vi "Test-Motors with Encoders-Report Motor State.vi"() -> ()   [LabVIEW 2014, in "Comp Motors with Encoders.lvlib"]
uses:
  Comp Motors with Encoders.lvlib
  Robot Actor Framework/Trace/Trace Controller Class/Config.ctl
  Robot/Joystick/Joystick Class/Joystick State.ctl
  Robot/Joystick/Joystick Class/Button State.ctl
  Robot/Joystick/Joystick Class/Axis State.ctl
  Comp Xbox One Controller/Comp XBox One Controller Class/Comp X1 Config.ctl
  <vilib>/Rock Robotics/WPI/Joystick/WPI_JoystickDeviceEnum.ctl
  Comp Trace Controller/Comp Trace Controller Class/Comp Trace Controller.lvclass
  Comp Pressure/Comp Pressure Class/Comp Pressure.lvclass
  Comp Xbox One Controller/Comp XBox One Controller Class/Comp XBox One Controller.lvclass
  Comp Xbox One Controller/Test-XBox Controller-Receive Updates/Test-XBox Controller-Receive Updates.lvclass
  Comp Xbox One Controller/Comp XBox One Controller Class/Comp XBox One Controller.lvclass/Comp XBox One Controller.ctl
  <vilib>/Rock Robotics/WPI/DriverStation/WPI_DriverStationRobotMode2.ctl
  Comp Xbox One Controller/Test-XBox Controller-Receive Updates Messages/Receive Joystick Update Msg/Receive Joystick Update Msg.lvclass
  Robot/Joystick/Joystick Messages/Request Joystick State Msg/Request Joystick State Msg.lvclass/Request Joystick State Msg.ctl
  <vilib>/ActorFramework/Message Enqueuer/Message Enqueuer.lvclass/Message Enqueuer.ctl
  <vilib>/ActorFramework/Message Enqueuer/Enqueue.vi
  <vilib>/ActorFramework/Message Priority Queue/Priority Enqueue.vi
  Robot/Joystick/Joystick Messages/Request Joystick State Msg/Request Joystick State Msg.lvclass
  <vilib>/ActorFramework/Stop Msg/Stop Msg.lvclass
  <vilib>/ActorFramework/Actor/Actor.lvclass
  Robot Actor Framework/Trace/Trace Controller Class/Trace Controller.lvclass
  Robot/Joystick/Joystick Class/Joystick.lvclass
panel:
  in  "XBox One Controller Config":T1={"Joystick USB"=enum."USB 0", "Deadband"=0.1}
  in  "Joystick State":T3
  in  "Test Loop":u32=75
  out "Enable Tele":bool caption="Enabled Teleop"
  in  "Stop Test Loop 1":bool=TRUE
  in  "Finish Test":bool=TRUE
  in  "Start Test":bool=TRUE
  in  "Trace Controller Config":T6={"Folder Pattern"="/media/sd%s1", "Starting Letter Position"=1, "Min Free Space (MB)"=50.0, "Max Folders to Check"=10, "Trace Level"=enum."Debug"} {"Min Free Space (MB)" format="%#_13g"}
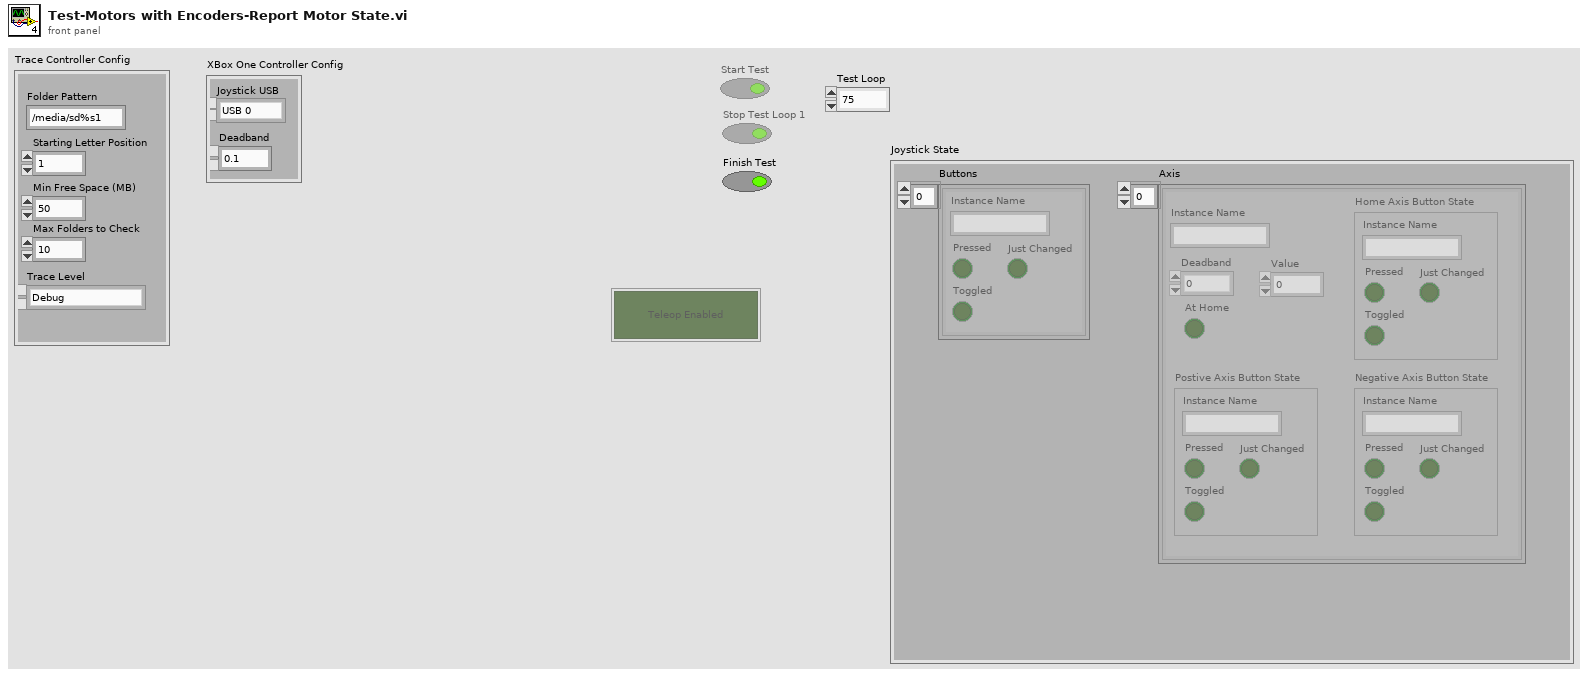
[diagram p1: front panel]
types:
  T1 = typedef "Comp XBox One Controller.lvlib/Comp XBox One Controller.lvclass/Comp X1 Config.ctl" = cluster{"Joystick USB":T2, "Deadband":dbl}
  T2 = typedef "WPI_JoystickDeviceEnum.ctl" = enum16{"USB 0", "USB 1", "USB 2", "USB 3", "USB 4", "USB 5"}
  T3 = typedef "Joystick.lvlib/Joystick.lvclass/Joystick State.ctl" = cluster{"Buttons":T4[], "Axis":T5[]}
  T4 = typedef "Joystick.lvlib/Joystick.lvclass/Button State.ctl" = cluster{"Pressed":bool, "Instance Name":string, "Toggled":bool, "Just Changed":bool}
  T5 = typedef "Joystick.lvlib/Joystick.lvclass/Axis State.ctl" = cluster{"Instance Name":string, "Deadband":dbl, "Value":dbl, "At Home":bool, "Postive Axis Button State":T4, "Negative Axis Button State":T4, "Home Axis Button State":T4}
  T6 = typedef "Robot Actor Framework.lvlib/Trace.lvlib/Trace Controller.lvclass/Config.ctl" = cluster{"Folder Pattern":string, "Starting Letter Position":i32, "Min Free Space (MB)":dbl, "Max Folders to Check":u32, "Trace Level":enum16{"Critical", "Error", "Warning", "Informational", "Debug"}}
  T7 = enum16{"Critical", "Error", "Warning", "Informational", "Debug"}
  T8 = enum8{"Enabled", "Disabled", "Disabled and Grayed Out"}
  T9 = typedef "WPI_DriverStationRobotMode2.ctl" = enum16{"Autonomous Disabled", "Autonomous Enabled", "Teleop Disabled", "Teleop Enabled", "Disconnected", "Finish", "Test Disabled", "Test Enabled", "Emergency Stopped"}
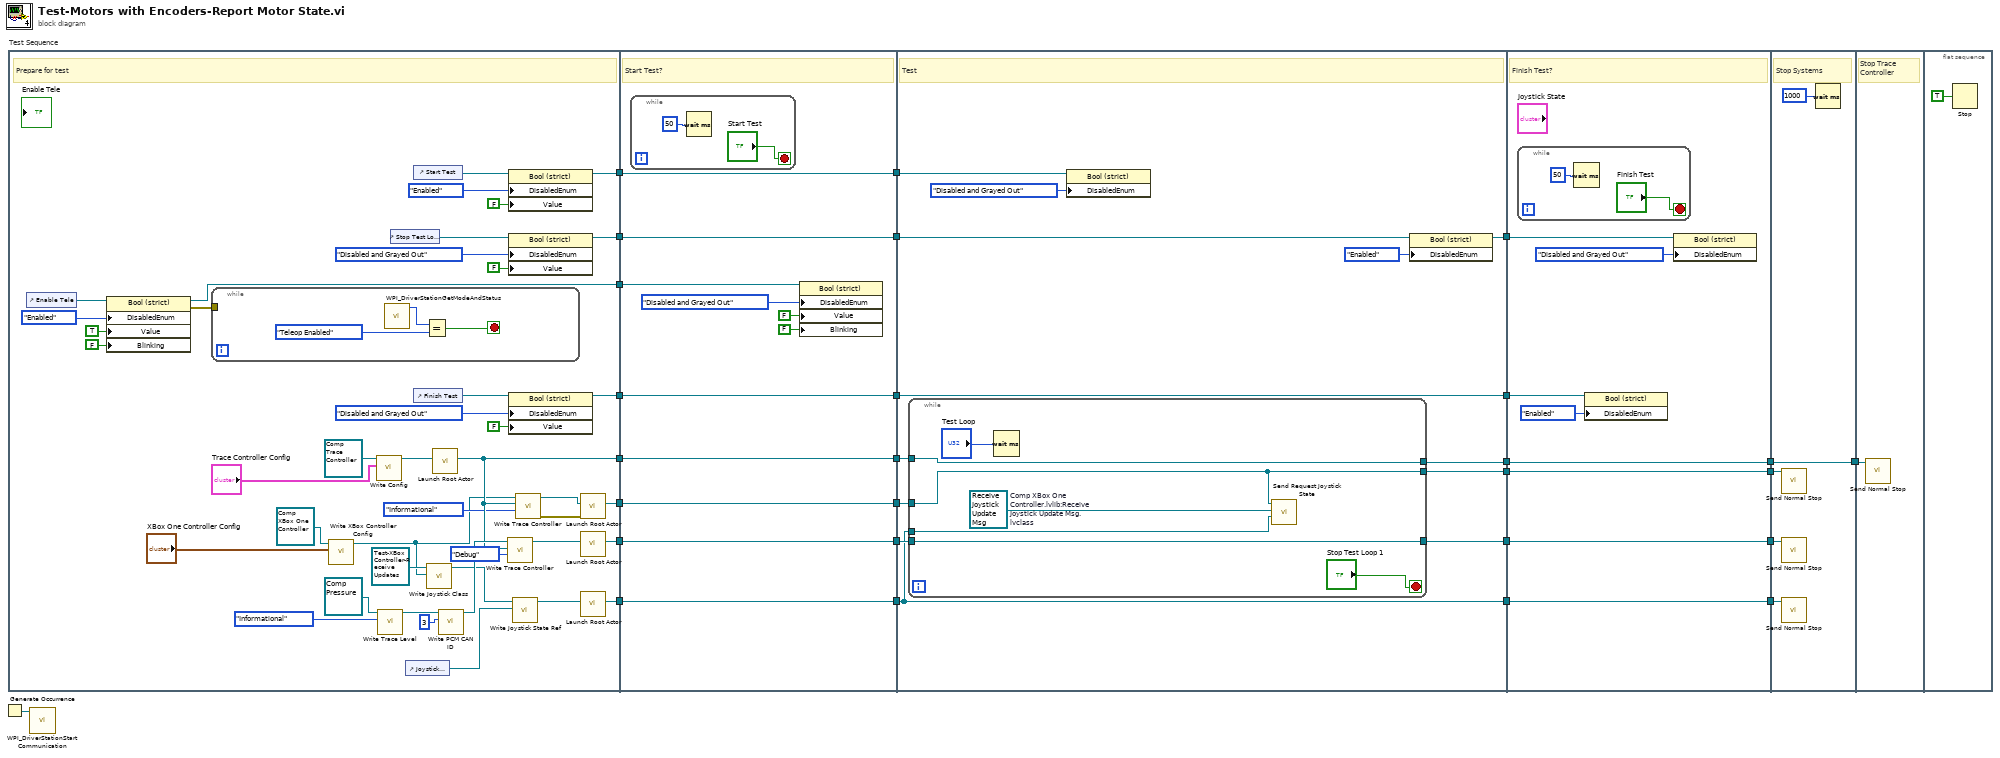
[diagram p0: block diagram]
diagram:
  n1 = Generate Occurrence() -> (w27:refnum<k4>)
  n2 = flat-sequence "Test Sequence" {
    tunnel: [w57] -> w16
    tunnel: [w59] -> w15
    tunnel: [w58] -> w14
    tunnel: [w47] -> w13
    tunnel: [w46] -> w11
    tunnel: [w45] -> w6
    tunnel: [w39] -> w5
    tunnel: [w29] -> w3
    tunnel: [w83] -> w19
    tunnel: [w82] -> w18
    tunnel: [w81] -> w17
    tunnel: w16 -> [w83]
    tunnel: w15 -> [w82]
    tunnel: w14 -> [w81]
    tunnel: w13 -> [w80]
    tunnel: [w80] -> w12
    tunnel: w11 -> [w79]
    tunnel: [w79] -> w10
    tunnel: [w78] -> w7
    tunnel: w6 -> [w78]
    tunnel: w5 -> [w77]
    tunnel: [w73] -> w4
    tunnel: w3 -> [w73]
    tunnel: [w93] -> w22
    tunnel: [w95] -> w21
    tunnel: [w94] -> w20
    tunnel: w19 -> [w98]
    tunnel: w18 -> [w96]
    tunnel: w17 -> [w97]
    tunnel: w12 -> [w92]
    tunnel: w10 -> [w90]
    tunnel: [w88] -> w9
    tunnel: [w87] -> w8
    tunnel: w7 -> [w87]
    tunnel: w4 -> [w86]
    tunnel: [w86] -> w2
    tunnel: [w113] -> w25
    tunnel: [w112] -> w24
    tunnel: [w111] -> w23
    tunnel: w22 -> [w113]
    tunnel: w21 -> [w112]
    tunnel: w20 -> [w111]
    tunnel: w9 -> [w110]
    tunnel: w8 -> [w107]
    tunnel: w2 -> [w106]
    tunnel: [w106] -> w1
    tunnel: [w120] -> w26
    tunnel: w25 -> [w120]
    tunnel: w24 -> [w119]
    tunnel: w23 -> [w117]
    tunnel: w1 -> [w116]
    tunnel: w26 -> [w121]
    frame #0 {
      # "Prepare for test"
      n3 = control-ref of="Enable Tele"() -> (w44:refnum<vi>)
      n4 = property class="Bool (strict)"(reference=w44, "DisabledEnum"=T8."Enabled" ("Disabled"), "Value"=TRUE, "Blinking"=FALSE) -> (reference out=w39:refnum<vi>, error out=w41:errorcluster)  [unwired: 1 in]
      n5 = while {
        tunnel: w41 -> [_]
        stop <- w70 stop-if-true
        n6 = call <vilib>:"WPI_DriverStationGetModeAndStatus.vi"() -> ("Robot Mode"=w72:T9)  [unwired: 10 in, 1 out]
        n7 = Equal?(x=w72, y=WPI_DriverStationRobotMode2."Teleop Enabled") -> (x = y?=w70:bool)
      }
      n8 = call "Write XBox Controller Config.vi"("XBox One Controller Config"="XBox One Controller Config", "Comp XBox One Controller in"=refnum<class "Comp XBox One Controller.lvclass"> refnum ("Comp XBox One Controller.lvlib:Comp XBox One Controller.lvclass")) -> ("Comp XBox One Controller out"=w31:refnum<class "Comp XBox One Controller.lvclass">)  [unwired: 8 in, 1 out]
      n9 = call-dynamic "Write Config.vi"("Config"="Trace Controller Config", "Trace Controller in"=refnum<class "Comp Trace Controller.lvclass"> refnum ("Comp Trace Controller.lvlib:Comp Trace Controller.lvclass")) -> ("Trace Controller out"=w62:refnum<class "Comp Trace Controller.lvclass">)  [unwired: 8 in, 1 out]
      n10 = call-dynamic "Write Trace Level.vi"("Trace Level"=T7."Informational", "System Actor in"=refnum<class "Comp Pressure.lvclass"> refnum ("Comp Pressure.lvlib:Comp Pressure.lvclass")) -> ("System Actor out"=w67:refnum<class "Comp Pressure.lvclass">)  [unwired: 8 in, 1 out]
      n11 = control-ref of="Stop Test Loop 1"() -> (w51:refnum<vi>)
      n12 = control-ref of="Joystick State"() -> (w33:refnum<vi>)
      n13 = control-ref of="Start Test"() -> (w56:refnum<vi>)
      n14 = control-ref of="Finish Test"() -> (w50:refnum<vi>)
      n15 = call-dynamic "Write Joystick Class.vi"("Joystick.lvlib:Joystick.lvclass"=w31, "Test-XBox Controller-Receive Updates in"=refnum<class "Test-XBox Controller-Receive Updates.lvclass"> refnum ("Comp XBox One Controller.lvlib:Test-XBox Controller-Receive Updates.lvclass")) -> ("Test-XBox Controller-Receive Updates out"=w34:refnum<class "Test-XBox Controller-Receive Updates.lvclass">)  [unwired: 8 in, 1 out]
      n16 = call <vilib>:"Launch Root Actor.vi"("Actor"=w62) -> ("Actor's Enqueuer"=w58:refnum<class "Message Enqueuer.lvclass">)  [unwired: 9 in, 1 out]
      n17 = call-dynamic "Write PCM CAN ID.vi"("PCM CAN ID"=u8 3, "Comp Pressure in"=w67) -> ("Comp Pressure out"=w68:refnum<class "Comp Pressure.lvclass">)  [unwired: 8 in, 1 out]
      n18 = call-dynamic "Write Trace Controller.vi"("Trace Level"=T7."Debug", "Trace Controller"=w58, "System Actor in"=w68) -> ("System Actor out"=w69:refnum<class "Comp Pressure.lvclass">)  [unwired: 7 in, 1 out]
      n19 = property class="Bool (strict)"(reference=w56, "DisabledEnum"=T8."Enabled" ("Disabled"), "Value"=FALSE) -> (reference out=w47:refnum<vi>)  [unwired: 1 in, 1 out]
      n20 = property class="Bool (strict)"(reference=w51, "DisabledEnum"=T8."Disabled and Grayed Out" ("Disabled"), "Value"=FALSE) -> (reference out=w46:refnum<vi>)  [unwired: 1 in, 1 out]
      n21 = property class="Bool (strict)"(reference=w50, "DisabledEnum"=T8."Disabled and Grayed Out" ("Disabled"), "Value"=FALSE) -> (reference out=w45:refnum<vi>)  [unwired: 1 in, 1 out]
      n22 = call-dynamic "Write Joystick State Ref.vi"("Joystick State Ref"=w33, "Test-XBox Controller-Receive Updates in"=w34) -> ("Test-XBox Controller-Receive Updates out"=w32:refnum<class "Test-XBox Controller-Receive Updates.lvclass">)  [unwired: 8 in, 1 out]
      n23 = call-dynamic "Write Trace Controller.vi"("Trace Level"=T7."Informational", "Trace Controller"=w58, "System Actor in"=w31) -> ("error out"=w64:errorcluster, "System Actor out"=w63:refnum<class "Comp XBox One Controller.lvclass">)  [unwired: 7 in]
      n24 = call <vilib>:"Launch Root Actor.vi"("error in (no error)"=w64, "Actor"=w63) -> ("Actor's Enqueuer"=w57:refnum<class "Message Enqueuer.lvclass">)  [unwired: 8 in, 1 out]
      n25 = call <vilib>:"Launch Root Actor.vi"("Actor"=w69) -> ("Actor's Enqueuer"=w59:refnum<class "Message Enqueuer.lvclass">)  [unwired: 9 in, 1 out]
      n26 = call <vilib>:"Launch Root Actor.vi"("Actor"=w32) -> ("Actor's Enqueuer"=w29:refnum<class "Message Enqueuer.lvclass">)  [unwired: 9 in, 1 out]
    }
    frame #1 {
      # "Start Test?"
      n27 = while {
        stop <- "Start Test" stop-if-true
        n28 = Wait (ms)(milliseconds to wait=u32 50) -> ()  [unwired: 1 out]
      }
      n29 = property class="Bool (strict)"(reference=w77, "DisabledEnum"=T8."Disabled and Grayed Out" ("Disabled"), "Value"=FALSE, "Blinking"=FALSE) -> ()  [unwired: 1 in, 2 out]
    }
    frame #2 {
      # "Test"
      n30 = while {
        tunnel: w97 -> [w104]
        tunnel: [w104] -> w93
        tunnel: w98 -> [w101]
        tunnel: [w101] -> w95
        tunnel: w96 -> [w103]
        tunnel: [w103] -> w94
        tunnel: w86 -> [w100]
        stop <- "Stop Test Loop 1" stop-if-true
        w99 = refnum<class "Receive Joystick Update Msg.lvclass"> refnum  # Comp XBox One Controller.lvlib:Receive Joystick Update Msg.lvclass
        n31 = Wait (ms)(milliseconds to wait="Test Loop") -> ()  [unwired: 1 out]
        n32 = call "Send Request Joystick State.vi"("Caller Enqueuer"=w100, "Joystick State Msg"=w99, "Message Enqueuer"=w101) -> ()  [unwired: 7 in, 2 out]
      }
      n33 = property class="Bool (strict)"(reference=w92, "DisabledEnum"=T8."Disabled and Grayed Out" ("Disabled")) -> ()  [unwired: 1 in, 2 out]
      n34 = property class="Bool (strict)"(reference=w90, "DisabledEnum"=T8."Enabled" ("Disabled")) -> (reference out=w88:refnum<vi>)  [unwired: 1 in, 1 out]
    }
    frame #3 {
      # "Finish Test?"
      n35 = while {
        stop <- "Finish Test" stop-if-true
        n36 = Wait (ms)(milliseconds to wait=u32 50) -> ()  [unwired: 1 out]
      }
      n37 = property class="Bool (strict)"(reference=w107, "DisabledEnum"=T8."Enabled" ("Disabled")) -> ()  [unwired: 1 in, 2 out]
      n38 = property class="Bool (strict)"(reference=w110, "DisabledEnum"=T8."Disabled and Grayed Out" ("Disabled")) -> ()  [unwired: 1 in, 2 out]
    }
    frame #4 {
      # "Stop Systems"
      n39 = call <vilib>:"Send Normal Stop.vi"("Message Enqueuer"=w119) -> ()  [unwired: 10 in, 1 out]
      n40 = call <vilib>:"Send Normal Stop.vi"("Message Enqueuer"=w117) -> ()  [unwired: 10 in, 1 out]
      n41 = call <vilib>:"Send Normal Stop.vi"("Message Enqueuer"=w116) -> ()  [unwired: 10 in, 1 out]
      n42 = Wait (ms)(milliseconds to wait=u32 1000) -> ()  [unwired: 1 out]
    }
    frame #5 {
      # "Stop Trace Controller"
      n43 = call <vilib>:"Send Normal Stop.vi"("Message Enqueuer"=w121) -> ()  [unwired: 10 in, 1 out]
    }
    frame #6 {
      n44 = Stop(stop? (T)=TRUE) -> ()
    }
  }
  n45 = call <vilib>:"WPI_DriverStationStart Communication.vi"("occurrence"=w27) -> ()  [unwired: 1 in, 10 out]
